vi "DestroyWindow.vi"(8 "error in (no error)":errorcluster, 11 "Window in":refnum<class "Window.lvclass">) -> (0 "error out":errorcluster, 3 "Window out":refnum<class "Window.lvclass">)   [LabVIEW 2024, in "GLF.lvlib" / "Window.lvclass"]
uses:
  Window.lvclass
  Window.lvclass/Window.ctl
  <vilib>/Saukko/LV SDL3/Sources/SDL3/Video/Video.lvlib
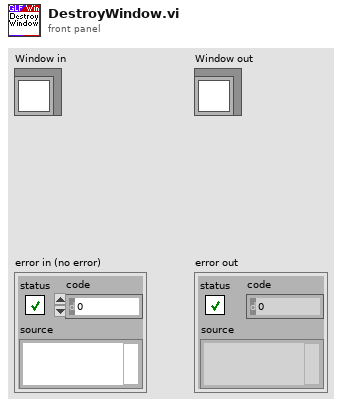
[diagram p1: front panel]
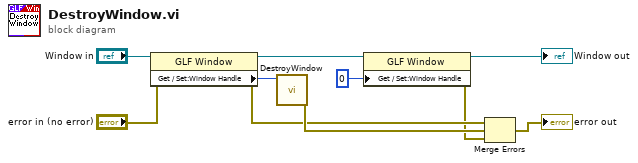
[diagram p0: block diagram]
diagram:
  n1 = property class="GLF Window"(reference="Window in", error in="error in (no error)") -> (reference out=w8:refnum<class "Window.lvclass">, error out=w6:errorcluster, "Get / Set:Window Handle"=w4:i64)
  n2 = call <vilib>:"DestroyWindow.vi"("Window [SDL_Window*]"=w4) -> ("Error Out"=w9:errorcluster)  [unwired: 10 in]
  n3 = property class="GLF Window"(reference=w8, "Get / Set:Window Handle"=i64 0 ("SDL_Window *")) -> (reference out=→"Window out":refnum<class "Window.lvclass">, error out=w1:errorcluster)  [unwired: 1 in]
  n4 = Merge Errors(w6, w9, w1) -> (→"error out":errorcluster)
